vi "Command_DrivePath.vi"(0 "Name of Path":string, 7 "Parameters":dbl[](array[numeric])=[60.0, 180.0, 2.0, 0.5, 10.0], 11 "Startup":bool) -> (4 "Completed":bool=TRUE, 6 "Drive_Motor_Values":dbl[](array[numeric]), 10 "Azimuth_Motor_Values":dbl[](array[numeric]), 15 "Reinit":bool)   [LabVIEW 2020]
uses:
  Auto Utilities/Command_Execution_State.ctl
  Globals/Sensor_Values.vi
  <vilib>/Utility/file.llb/Read Delimited Spreadsheet (DBL).vi
  Globals/FilePath_Globals.vi
panel:
  in  "PID Drive Tuning":T1={"Kp"=0.0001, "Ki"=0.0, "Kd"=0.0, "N-Diff"=10, "N-Int"=20, "Int Error Window"=0.5, "Max Ouput"=1.0, "Min Output"=-1.0} {"Int Error Window" min=0.0; "N-Int" min=2; "N-Diff" min=2; "Kd" min=0.0; "Ki" min=0.0; "Kp" min=0.0}
  in  "PID Heading Tuning":T1={"Kp"=0.0005, "Ki"=0.0, "Kd"=0.0, "N-Diff"=10, "N-Int"=20, "Int Error Window"=0.5, "Max Ouput"=1.0, "Min Output"=-1.0} {"Int Error Window" min=0.0; "N-Int" min=2; "N-Diff" min=2; "Kd" min=0.0; "Ki" min=0.0; "Kp" min=0.0}
  in  "Plot?":bool
  out "PID Heading":T2(graph)={"Command"=0.0, "Proportional"=-0.0, "Integral"=0.0, "Derivative"=0.0, "Goal"=0.0}
  out "PID Drive":T2(graph)
  out "Path and Robot Pose":cluster{dbl[], dbl[]}[](graph)
  out "Distance from End (in)":dbl=0.2721783737612782
  out "Distance from Start (in)":dbl=311.9984800663311
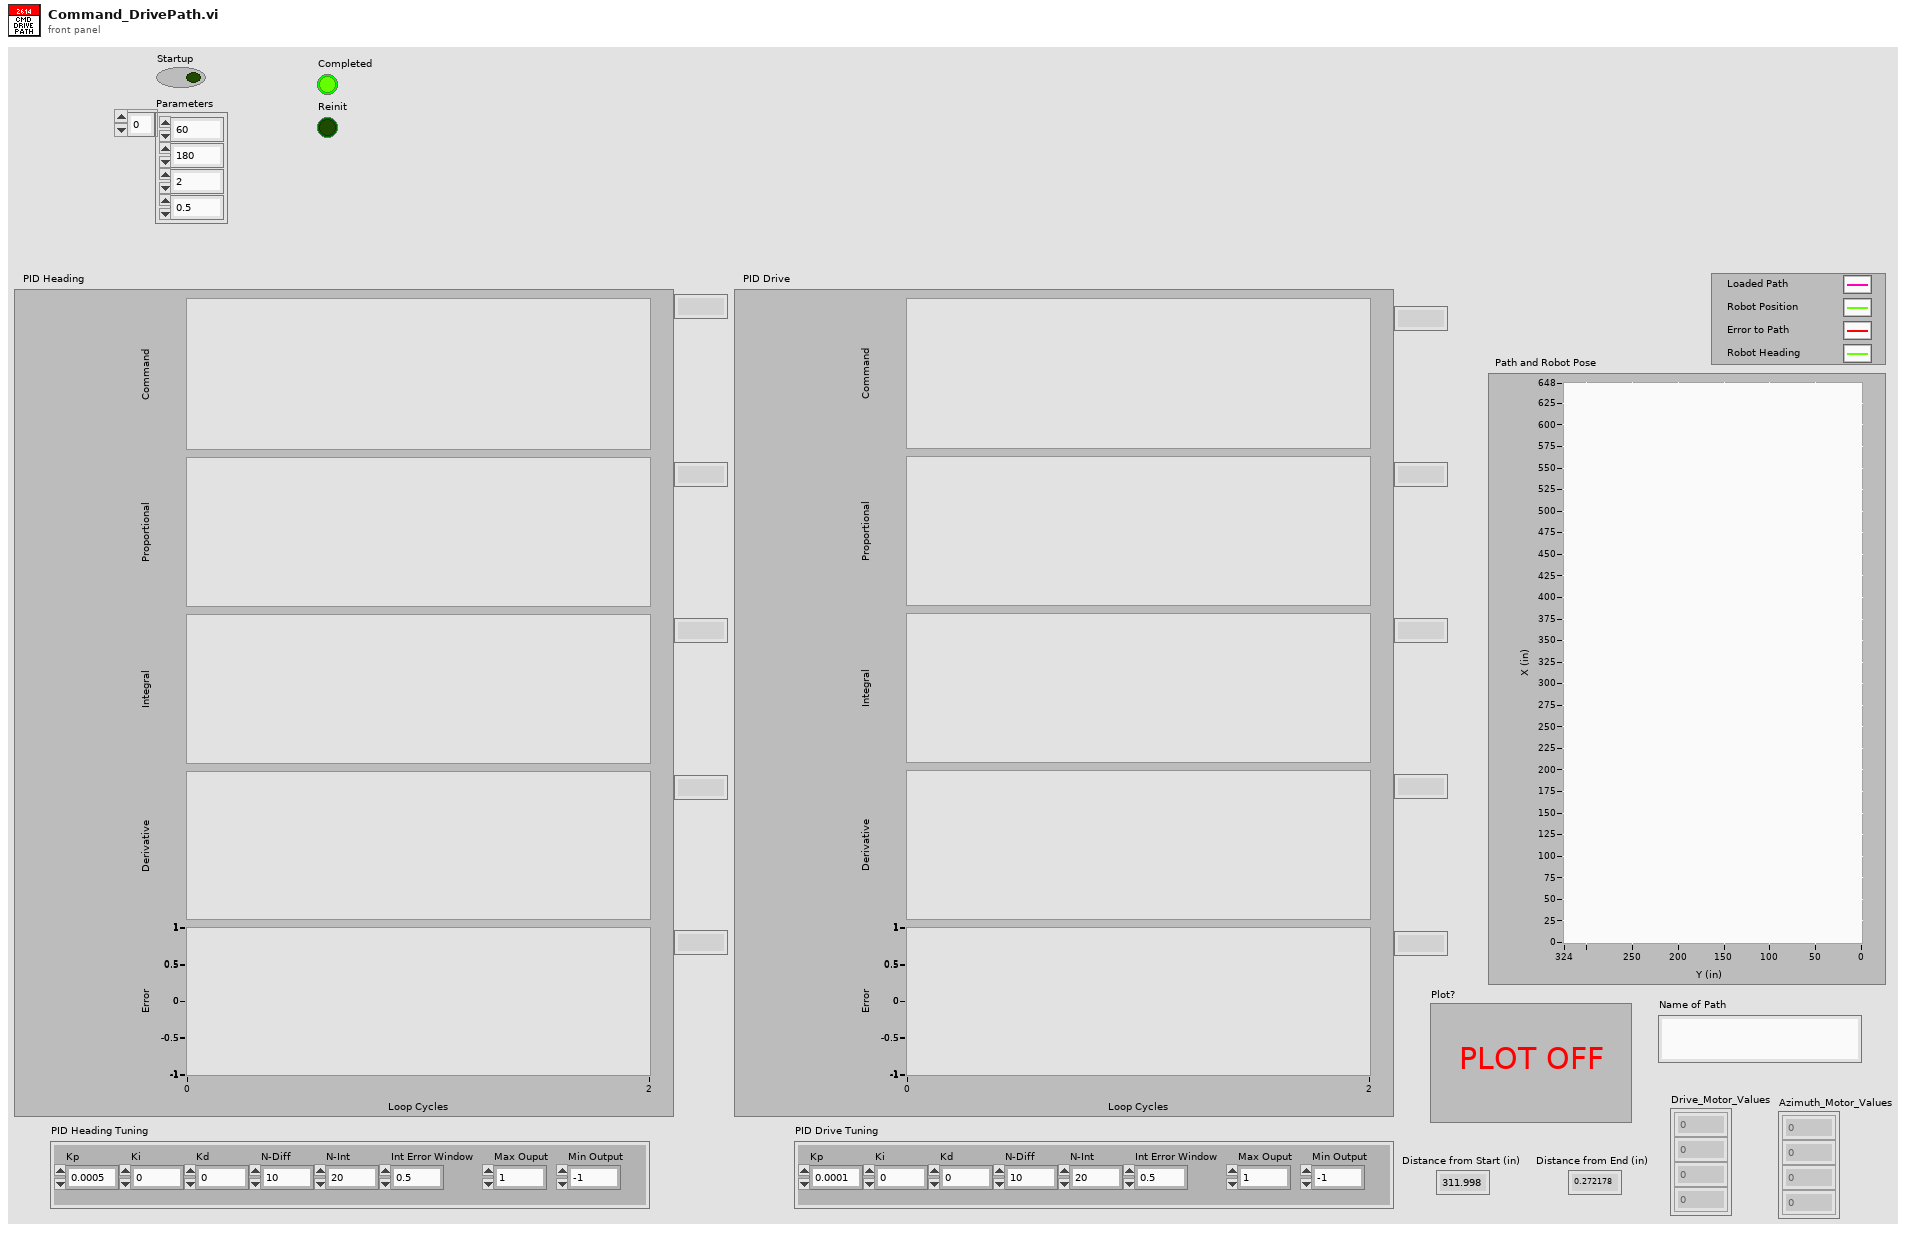
[diagram p1: front panel]
types:
  T1 = cluster{"Kp":dbl, "Ki":dbl, "Kd":dbl, "N-Diff":i32, "N-Int":i32, "Int Error Window":dbl, "Max Ouput":dbl, "Min Output":dbl}
  T2 = cluster{"Command":dbl, "Proportional":dbl, "Integral":dbl, "Derivative":dbl, "Goal":dbl}
  T3 = typedef "Command_Execution_State.ctl" = enum16{"Initialize", "Execute", "Finish"}
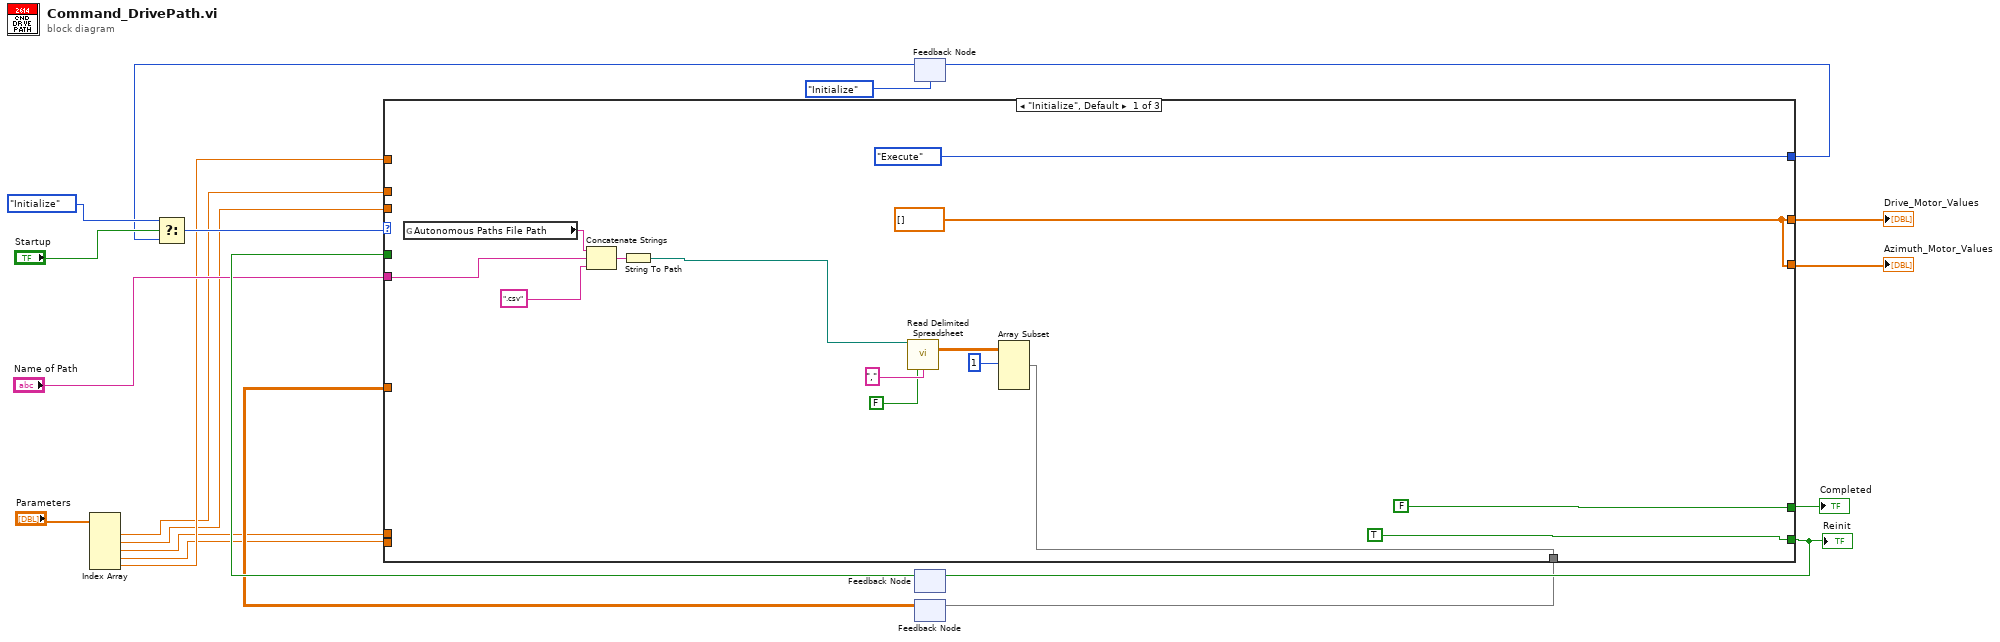
[diagram p0: block diagram]
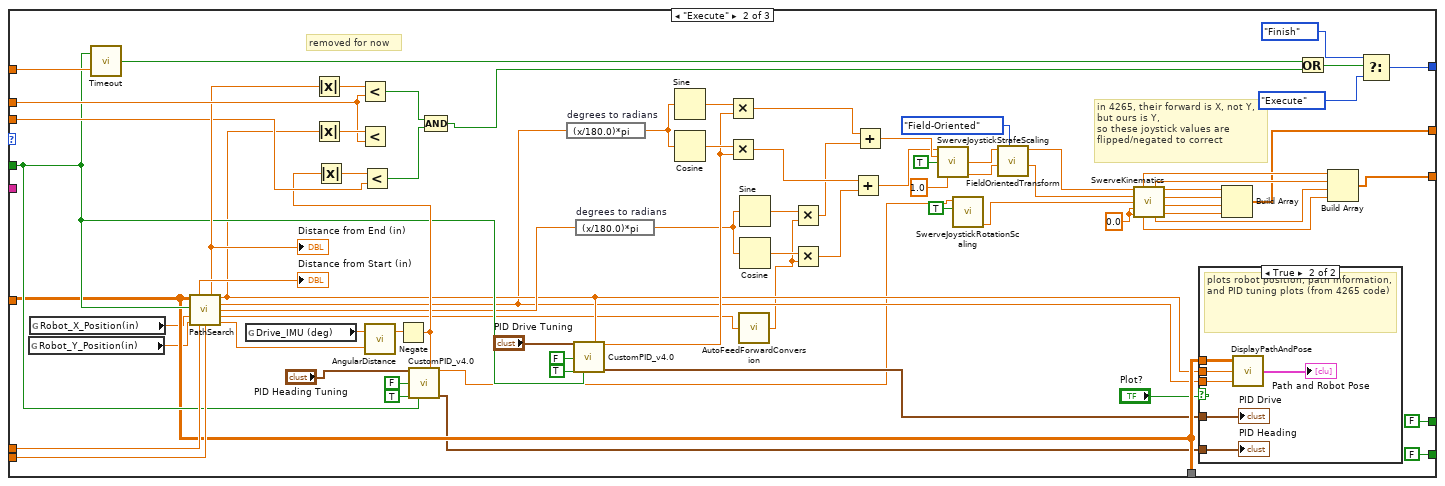
[diagram p2: hidden frame]
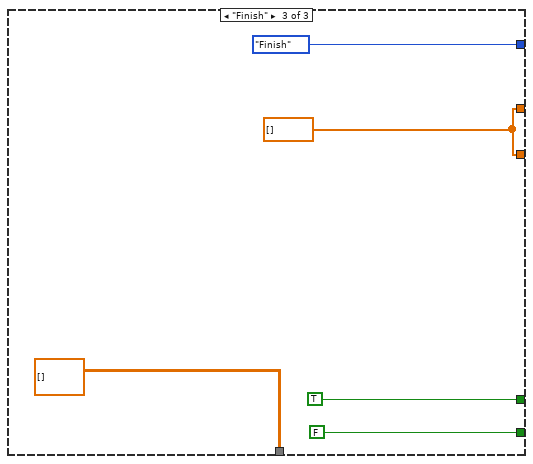
[diagram p4: hidden frame]
diagram:
  n1 = Index Array(array="Parameters") -> (element #1=w2:dbl, element #2=w1:dbl, element #3=w4:dbl, element #4=w3:dbl, element #5=w5:dbl)  [unwired: 5 in]
  n2 = feedback #1(Command_Execution_State."Initialize") -> (w16:T3)
  n3 = Select(t=Command_Execution_State."Initialize", s="Startup", f=w16) -> (s? t:f=w18:T3)
  n4 = feedback #2() -> (w12:bool)  [unwired: 1 in]
  n5 = feedback #3() -> (w6:dbl[][])  [unwired: 1 in]
  n6 = case shown="\"Initialize\", Default" w18 {
    tunnel: [Command_Execution_State."Execute" w108 Command_Execution_State."Finish"] -> w17
    tunnel: [FALSE ("Reinit") FALSE ("Reinit") TRUE ("Reinit")] -> w14
    tunnel: [TRUE ("Reinit") FALSE ("Reinit") FALSE ("Reinit")] -> w13
    tunnel: w12 -> [_ w85 _]
    tunnel: [w31 w61 w118] -> w11
    tunnel: [w31 w62 w118] -> w10
    tunnel: w5 -> [_ w103 _]
    tunnel: "Name of Path" -> [w27 _ _]
    tunnel: [w22 w84 dbl[][] [] ("Data (index by row)")] -> w7
    tunnel: w6 -> [_ w84 _]
    tunnel: w4 -> [_ w102 _]
    tunnel: w3 -> [_ w101 _]
    tunnel: w2 -> [_ w96 _]
    tunnel: w1 -> [_ w94 _]
    frame "Initialize", Default {
      w31 = dbl[] [] ("Drive_Motor_Values")
      n7 = global read "FilePath_Globals.vi" "Autonomous Paths File Path"() -> (w21:string)
      n8 = Concatenate Strings(w21, w27, ".csv" ("string")) -> (w29:string)
      n9 = String To Path(string=w29) -> (path=w28:path)
      n10 = call-poly <vilib>:"Read Delimited Spreadsheet.vi"("file path (dialog if empty)"=w28, "transpose? (F)"=FALSE, "delimiter (\\t)"="," ("delimiter (\\t)")) -> ("all rows"=w24:dbl[][])  [unwired: 7 in, 5 out]
      n11 = Array Subset(array=w24, index (row)=1 ("index")) -> (w22:dbl[][])  [unwired: 3 in]
    }
    frame "Execute" {
      w75 = 0.0 ("Cy (in)")
      # "removed for now"
      # "in 4265, their forward is X, not Y, but ours is Y,\nso these joystick values are flipped/negated to correct"
      n12 = global read "Sensor_Values.vi" "Robot_Y_Position(in)"() -> (w50:dbl)
      n13 = global read "Sensor_Values.vi" "Robot_X_Position(in)"() -> (w51:dbl)
      n14 = call "Timeout.vi"("Timeout"=w103, "Initialize"=w85) -> ("Timed Out?"=w104:bool)
      n15 = call "PathSearch.vi"("Path"=w84, "Reint"=w85, "Robot X (in)"=w51, "Robot Y (in)"=w50, "Search Window (s)"=w102, "Look-Ahead Time (s)"=w101) -> ("Distance from Start (in)"=→"Distance from Start (in)":dbl, "Distance from End (in)"=w95:dbl, "Feed Back Distance Error (in)"=w55:dbl, "Feed Back Pointing Angle (deg)"=w54:dbl, "Feed Forward Pointing Angle (deg)"=w79:dbl, "Feed Forward Velocity (in/s)"=w53:dbl, "Robot Heading Goal (deg)"=w93:dbl)  [unwired: 3 in]
      "Distance from End (in)" <- w95
      n16 = global read "Sensor_Values.vi" "Drive_IMU (deg)"() -> (w92:dbl)
      n17 = Absolute Value(x=w95) -> (abs(x)=w99:dbl)
      n18 = Absolute Value(x=w55) -> (abs(x)=w98:dbl)
      n19 = Less?(x=w99, y=w96) -> (x < y?=w38:bool)
      n20 = Less?(x=w98, y=w96) -> ()  [unwired: 1 out]
      n21 = call "AngularDistance.vi"("Goal Angle (deg) [0,360]"=w93, "Current Angle (deg) [-Inf,+Inf]"=w92) -> ("Signed Angular Distance (deg) [-180,+180]"=w91:dbl)  [unwired: 1 out]
      n22 = Negate(x=w91) -> (-x=w90:dbl)
      n23 = Absolute Value(x=w90) -> (abs(x)=w97:dbl)
      n24 = Less?(x=w97, y=w94) -> (x < y?=w37:bool)
      n25 = call "CustomPID_v4.0.vi"("PID Tuning Parameters"="PID Heading Tuning", "Custom Error Calculation"=w90, "Reset on Goal Change ?"=FALSE, "Use Custom Error Calculation ?"=TRUE, "Reinit"=w85) -> ("Command"=w41:dbl, "Controller Summary"=w57:T2)  [unwired: 7 in, 2 out]
      n26 = Compound Arithmetic op=AND(w38, w37) -> (w36:bool)
      n27 = expression code="(x/180.0)*pi" "degrees to radians"(w54) -> (w81:dbl)
      n28 = call "CustomPID_v4.0.vi"("PID Tuning Parameters"="PID Drive Tuning", "Custom Error Calculation"=w55, "Reset on Goal Change ?"=FALSE, "Use Custom Error Calculation ?"=TRUE, "Reinit"=w85) -> ("Command"=w80:dbl, "Controller Summary"=w58:T2)  [unwired: 7 in, 2 out]
      n29 = expression code="(x/180.0)*pi" "degrees to radians"(w79) -> (w76:dbl)
      n30 = Sine(x=w81) -> (sin(x)=w82:dbl)
      n31 = Cosine(x=w81) -> (cos(x)=w83:dbl)
      n32 = Multiply(x=w82, y=w80) -> (x*y=w72:dbl)
      n33 = Multiply(x=w83, y=w80) -> (x*y=w73:dbl)
      n34 = call "AutoFeedForwardConversion.vi"("Target Velocity (in/s)"=w53) -> ("Equivalent Joystick Command (ul)"=w52:dbl)
      n35 = Sine(x=w76) -> (sin(x)=w78:dbl)
      n36 = Cosine(x=w76) -> (cos(x)=w77:dbl)
      n37 = Multiply(x=w78, y=w52) -> (x*y=w71:dbl)
      n38 = Multiply(x=w77, y=w52) -> (x*y=w74:dbl)
      n39 = Add(x=w73, y=w74) -> (x+y=w48:dbl)
      n40 = Add(x=w72, y=w71) -> (x+y=w49:dbl)
      n41 = call "SwerveJoystickStrafeScaling.vi"("Raw Joystick X"=w48, "Raw Joystick Y"=w49, "Auto Control"=TRUE, "Strafe Maximum"=1.0) -> ("Scaled Joystick X"=w46:dbl, "Scaled Joystick Y"=w45:dbl)  [unwired: 9 in, 1 out]
      n42 = call "SwerveJoystickRotationScaling.vi"("Auto Control"=TRUE, "Raw Joystick Rotation"=w41) -> ("Scaled Joystick Rotation"=w39:dbl)  [unwired: 7 in, 1 out]
      n43 = call "FieldOrientedTransform.vi"("Orientation Mode"=enum16{"Robot-Oriented", "Field-Oriented"}."Field-Oriented", "Joystick Y"=w45, "Joystick X"=w46) -> ("Joystick Y'"=w42:dbl, "Joystick X'"=w43:dbl)  [unwired: 7 in]
      n44 = call "SwerveKinematics.vi"("Joystick X"=w43, "Joystick Y"=w42, "Joystick Rotation"=w39, "Cx (in)"=w75, "Cy (in)"=w75) -> ("Module 0 Angle (deg)"=w66:dbl, "Module 1 Angle (deg)"=w65:dbl, "Module 0 Velocity Command (ul)"=w70:dbl, "Module 1 Velocity Command (ul)"=w69:dbl, "Module 2 Velocity Command (ul)"=w68:dbl, "Module 3 Angle (deg)"=w63:dbl, "Module 2 Angle (deg)"=w64:dbl, "Module 3 Velocity Command (ul)"=w67:dbl)  [unwired: 3 in]
      n45 = case shown="True" "Plot?" {
        tunnel: w84 -> [_ w116]
        tunnel: w54 -> [_ w115]
        tunnel: w55 -> [_ w114]
        tunnel: w58 -> [_ w113]
        tunnel: w57 -> [_ w112]
        frame False {
        }
        frame True {
          # "plots robot position, path information, and PID tuning plots (from 4265 code)"
          n46 = call "DisplayPathAndPose.vi"("Feed Back Pointing Angle (deg)"=w115, "Feed Back Distance Error (in)"=w114, "Data (index by row)"=w116) -> ("Path and Robot Pose"=→"Path and Robot Pose":cluster{dbl[], dbl[]}[])
          "PID Drive" <- w113
          "PID Heading" <- w112
        }
      }
      n47 = Build Array(w70, w69, w68, w67) -> (w61:dbl[])
      n48 = Or(x=w104, y=w36) -> (x .or. y?=w105:bool)
      n49 = Build Array(w66, w65, w64, w63) -> (w62:dbl[])
      n50 = Select(t=Command_Execution_State."Finish", s=w105, f=Command_Execution_State."Execute") -> (s? t:f=w108:T3)
    }
    frame "Finish" {
      w118 = dbl[] [] ("Drive_Motor_Values")
    }
  }
  "Reinit" <- w13
  "Completed" <- w14
  "Drive_Motor_Values" <- w11
  "Azimuth_Motor_Values" <- w10
  n51 = feedback-in #1(w17) -> ()
  n52 = feedback-in #2(w13) -> ()
  n53 = feedback-in #3(w7) -> ()
